vi "1 Channel N Samples - Auto Indexing.vi"() -> ()   [LabVIEW 2026, in "synnax_clib.lvlib"]
uses:
  lvlib/synnax_clib.lvlib
  lvlib/typedefs/connection_config.ctl
  lvlib/classes/Client/Private/synnax channel retrieve keys Single.vi
  lvlib/classes/Writer/Private/synnax writer open Single.vi
  lvlib/classes/Writer/Private/Writes/DBL/Write 1Ch NSamp (DBL).vi
  lvlib/classes/Synnax Writer.lvclass
  lvlib/classes/Client/Synnax Client.lvclass
panel:
  in  "Channel":string="my_f64_chan"
  in  "Stop":bool
  out "error out":errorcluster
  in  "Connection Config":T1={"host"="localhost", "port"=9090, "username"="synnax", "password"="seldon"}
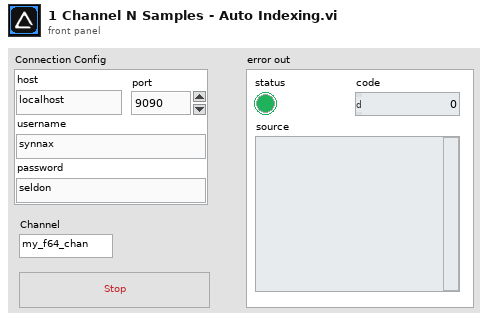
[diagram p1: front panel]
types:
  T1 = typedef "synnax_clib.lvlib/connection_config.ctl" = cluster{"host":string, "port":u16, "username":string, "password":string}
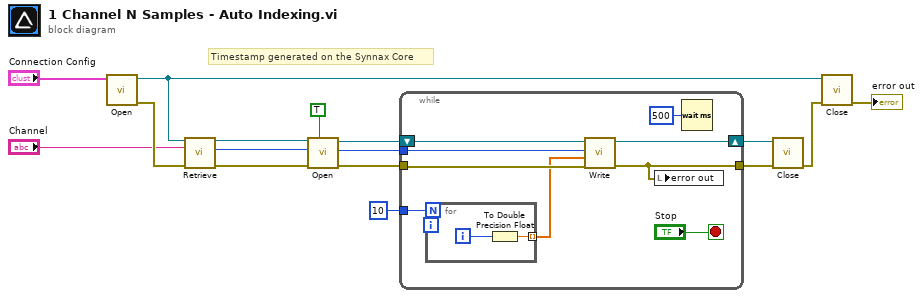
[diagram p0: block diagram]
diagram:
  # "Timestamp generated on the Synnax Core"
  n1 = call "Open.vi"("Connection Config"="Connection Config") -> ("error out"=w11:errorcluster, "Synnax Client out"=w13:refnum<class "Synnax Client.lvclass">)  [unwired: 9 in]
  n2 = call-poly "Retrieve.vi"("Synnax Client in"=w13, "channel name"="Channel", "error in"=w11) -> ("Synnax Client out"=w7:refnum<class "Synnax Client.lvclass">, "channel key"=w4:u32, "error out"=w15:errorcluster)  [unwired: 8 in, 2 out]
  n3 = call-poly "Open.vi"("auto_index (F)"=TRUE, "error in"=w15, "channel in"=w4, "Synnax Client in"=w7) -> ("error out"=w8:errorcluster, "channel out"=w2:u32, "writer out"=w10:refnum<class "Synnax Writer.lvclass">)  [unwired: 5 in]
  n4 = while {
    shift-right: [w24] -> w9
    shift-left: w10 -> [w25]
    tunnel: w8 -> [w23]
    tunnel: [w20] -> w16
    tunnel: 10 -> [w19]
    tunnel: w2 -> [w17]
    stop <- "Stop" stop-if-true
    n5 = for {
      N: w19 -> [_]
      tunnel: [w26] -> w21 mode=indexing
      i -> [w27]
      n6 = To Double Precision Float(number=w27) -> (double precision float=w26:dbl)
    }
    n7 = call-poly "Write.vi"("error in"=w23, "data"=w21, "channel"=w17, "Writer"=w25) -> ("error out"=w20:errorcluster, "Writer Out"=w24:refnum<class "Synnax Writer.lvclass">)  [unwired: 6 in]
    n8 = local write "error out"(w20) -> ()
    n9 = Wait (ms)(milliseconds to wait=u32 500) -> ()  [unwired: 1 out]
  }
  n10 = call "Close.vi"("error in"=w16, "writer"=w9) -> ("error out"=w12:errorcluster)  [unwired: 9 in]
  n11 = call "Close.vi"("error in"=w12, "Synnax Client in"=w13) -> ("error out"=→"error out":errorcluster)  [unwired: 9 in]
